vi "control loop bookkeeping.vi"(6 "worker pool reference":T2, 8 "engine error in":errorcluster, 9 "status reporting in":T18={"late? index (bool)"=-1, "late count index (U32)"=-1, "dt (ns) index (U64)"=-1}, 10 "time data in":T1, 11 "control loop data in":T5 {"module information"."GUID"."Lo" format="%.0x"; "module information"."GUID"."Hi" format="%.0x"}) -> (0 "engine error out":errorcluster, 1 "safe state?":bool, 2 "time data out":T1, 3 "control loop data out":T5 {"module information"."GUID"."Lo" format="%.0x"; "module information"."GUID"."Hi" format="%.0x"})   [LabVIEW 2013, in "main engine.lvlib"]
doc: "This VI writes to any of the timing or error tags that have been configured based on the results of this iteration of the loop."
uses:
  main engine.lvlib
  status reporting data.ctl
  control loop data.ctl
  <vilib>/NI/Tag Bus/table/data table.ctl
  engine run schedule.ctl
  engine decimation schedule.ctl
  full module data.ctl
  <vilib>/NI/Tag Bus Module Framework/runtime/TBM module execution interface.lvclass
  module run state.ctl
  async executor/asynchronous executor reference.ctl
  async executor/message to executor.ctl
  Runtime/async command notification.ctl
  Runtime/async error info.ctl
  <vilib>/NI/Tag Bus Module Framework/runtime/error classification.ctl
  <vilib>/NI/Tag Bus Module Framework/module configuration/TBM module configuration.lvclass
  <vilib>/NI/Configuration Framework/serializable configuration/Numeric GUID.ctl
  module method data.ctl
  <vilib>/NI/Tag Bus/table/transfer specification.ctl
  <vilib>/NI/Tag Bus/tag/Data Type.ctl
  fault handling spec.ctl
  Configuration/Error Actions.ctl
  worker library/worker comms.ctl
  worker library/worker commands.ctl
  worker library/request fifos.ctl
  worker library/recovery request.ctl
  worker library/rt fault.ctl
  worker library/response fifos.ctl
  worker library/recovery response.ctl
  <vilib>/NI/Module Execution Interface/Engine Runtime/Fault.ctl
  time information.ctl
  <vilib>/NI/Tag Bus/table/write data element.vi
  <vilib>/NI/Tag Bus/table/data polymorphs/write one/write I32.vi
  perform asynchronous fault handling.vi
  perform fault handling.vi
  <vilib>/NI/Tag Bus/table/data polymorphs/write one/write Boolean.vi
  <vilib>/NI/Tag Bus/table/data polymorphs/write one/write U32.vi
  <vilib>/NI/Tag Bus/table/data polymorphs/write one/write U64.vi
  worker library/request recovery.vi
  worker library/request fault.vi
  rt swap object in dvr.vi
  <vilib>/NI/Tag Bus/table/data table.lvlib
  <vilib>/NI/Tag Bus/tag/tag descriptor.lvclass
  Configuration/Standard Engine Configuration.lvclass
  async executor/async executor.lvlib
  <vilib>/NI/Configuration Framework/serializable configuration/NISE_CEF_serializable configuration.lvclass
  worker library/worker pool.lvlib
  <vilib>/NI/Module Execution Interface/Engine Runtime/Engine Runtime Interface.lvclass
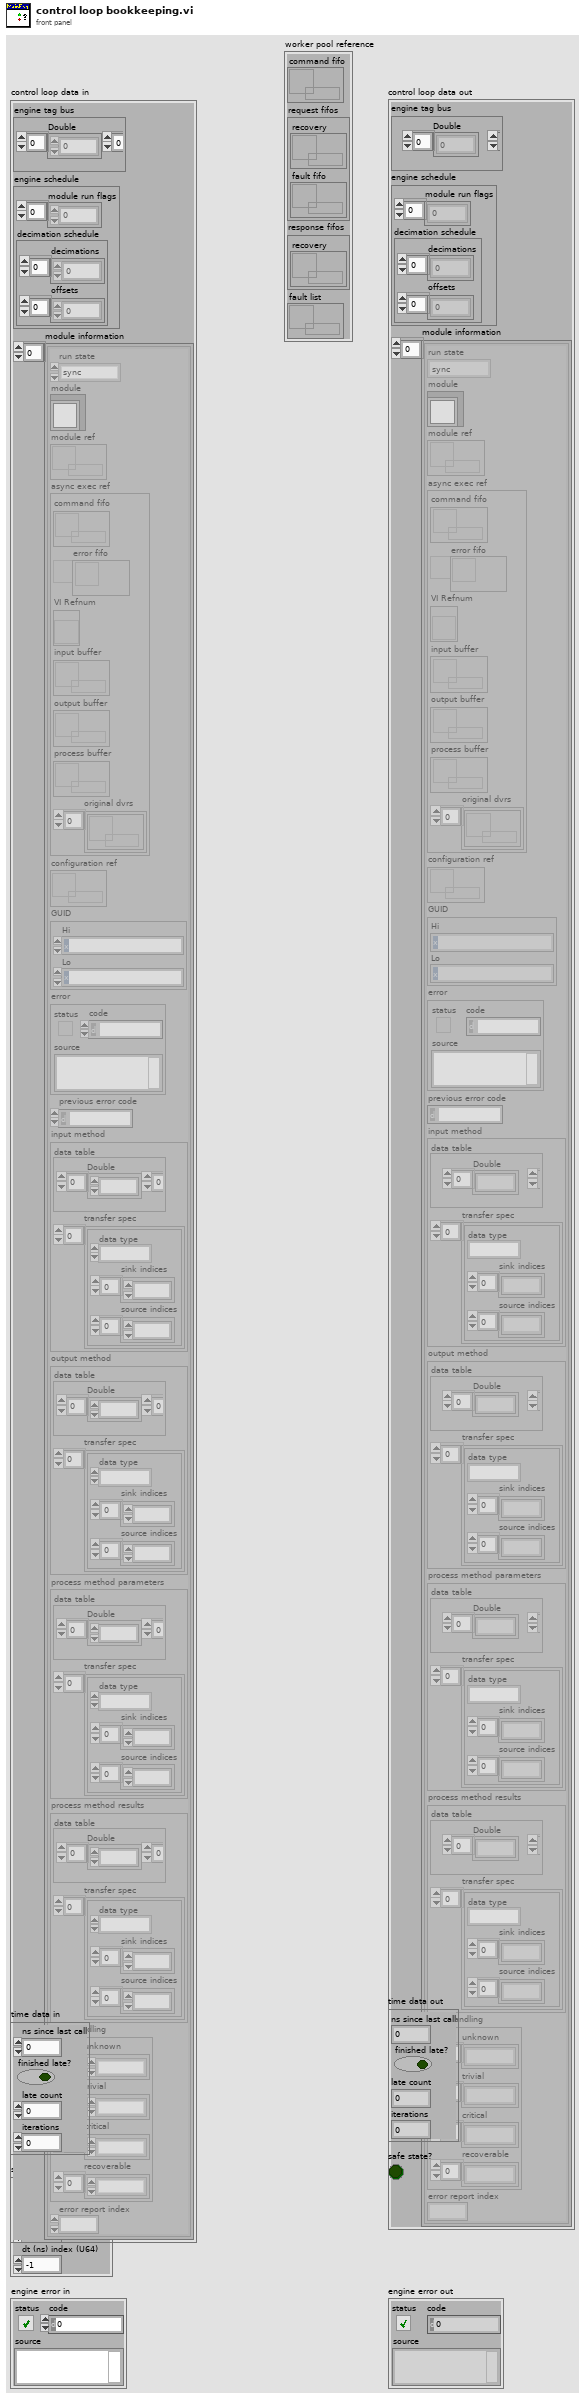
[diagram p1: front panel]
types:
  T1 = typedef "main engine.lvlib/time information.ctl" = cluster{"ns since last call":u64, "finished late?":bool, "late count":u32, "iterations":u64}
  T2 = typedef "worker pool.lvlib/worker comms.ctl" = cluster{"command fifo":refnum<k33>, "request fifos":T3, "response fifos":T4, "fault list":refnum<data-value>}
  T3 = typedef "worker pool.lvlib/request fifos.ctl" = cluster{"recovery":refnum<k33>, "fault fifo":refnum<k33>}
  T4 = typedef "worker pool.lvlib/response fifos.ctl" = cluster{"recovery":refnum<k33>}
  T5 = typedef "main engine.lvlib/control loop data.ctl" = cluster{"engine tag bus":T6, "engine schedule":T7, "module information":T9[]}
  T6 = typedef "tag bus.lvlib/data table.lvlib/data table.ctl" = cluster{"Double":dbl[], "Single":sgl[], "I64":i64[], "I32":i32[], "I16":i16[], "I8":i8[], "U64":u64[], "U32":u32[], "U16":u16[], "U8":u8[], "Boolean":bool[], "String":string[], "Array of Double":cluster{"DBL Array":dbl[]}[], "Array of Single":cluster{"SGL Array":sgl[]}[], "Array of I64":cluster{"I64 Array":i64[]}[], "Array of I32":cluster{"I32 Array":i32[]}[], "Array of I16":cluster{"I16 Array":i16[]}[], "Array of I8":cluster{"I8 Array":i8[]}[], "Array of U64":cluster{"U64 Array":u64[]}[], "Array of U32":cluster{"U32 Array":u32[]}[], "Array of U16":cluster{"U16 Array":u16[]}[], "Array of U8":cluster{"U8 Array":u8[]}[], "Array of Boolean":cluster{"Boolean Array":bool[]}[], "Array of String":cluster{"String Array":string[]}[]}
  T7 = typedef "main engine.lvlib/engine run schedule.ctl" = cluster{"module run flags":u8[], "decimation schedule":T8}
  T8 = typedef "main engine.lvlib/engine decimation schedule.ctl" = cluster{"decimations":u16[], "offsets":u16[]}
  T9 = typedef "main engine.lvlib/full module data.ctl" = cluster{"run state":T10, "module":refnum<class "TBM module execution interface.lvclass">, "module ref":refnum<data-value>, "async exec ref":T11, "configuration ref":refnum<data-value>, "GUID":T12, "error":errorcluster, "previous error code":i32, "input method":T13, "output method":T13, "process method parameters":T13, "process method results":T13, "fault handling":T16, "error report index ":i32}
  T10 = typedef "main engine.lvlib/module run state.ctl" = enum16{"sync", "async"}
  T11 = typedef "async executor.lvlib/asynchronous executor reference.ctl" = cluster{"command fifo":refnum<k33>, "error fifo":refnum<k33>, "VI Refnum":refnum<vi>, "input buffer":refnum<k33>, "output buffer":refnum<k33>, "process buffer":refnum<k33>, "original dvrs":refnum<data-value>[]}
  T12 = typedef "NISE_CEF_serializable configuration.lvclass/Numeric GUID.ctl" = cluster{"Hi":u64, "Lo":u64}
  T13 = typedef "main engine.lvlib/module method data.ctl" = cluster{"data table":T6, "transfer spec":T14[]}
  T14 = typedef "tag bus.lvlib/data table.lvlib/transfer specification.ctl" = cluster{"data type":T15, "sink indices":i32[], "source indices":i32[]}
  T15 = typedef "tag bus.lvlib/tag descriptor.lvclass/Data Type.ctl" = enum16{"Double", "Single", "I64", "I32", "I16", "I8", "U64", "U32", "U16", "U8", "Boolean", "String", "Array of Double", "Array of Single", "Array of I64", "Array of I32", "Array of I16", "Array of I8", "Array of U64", "Array of U32", "Array of U16", "Array of U8", "Array of Boolean", "Array of String"}
  T16 = typedef "main engine.lvlib/fault handling spec.ctl" = cluster{"unknown":T17[], "trivial":T17[], "critical":T17[], "recoverable":T17[]}
  T17 = typedef "Standard Engine Configuration.lvclass/Error Actions.ctl" = enum16{"Clear", "Notify", "Stop Component", "Stop Engine", "Safe State", "Attempt Recovery"}
  T18 = typedef "main engine.lvlib/status reporting data.ctl" = cluster{"late? index (bool)":i32, "late count index (U32)":i32, "dt (ns) index (U64)":i32}
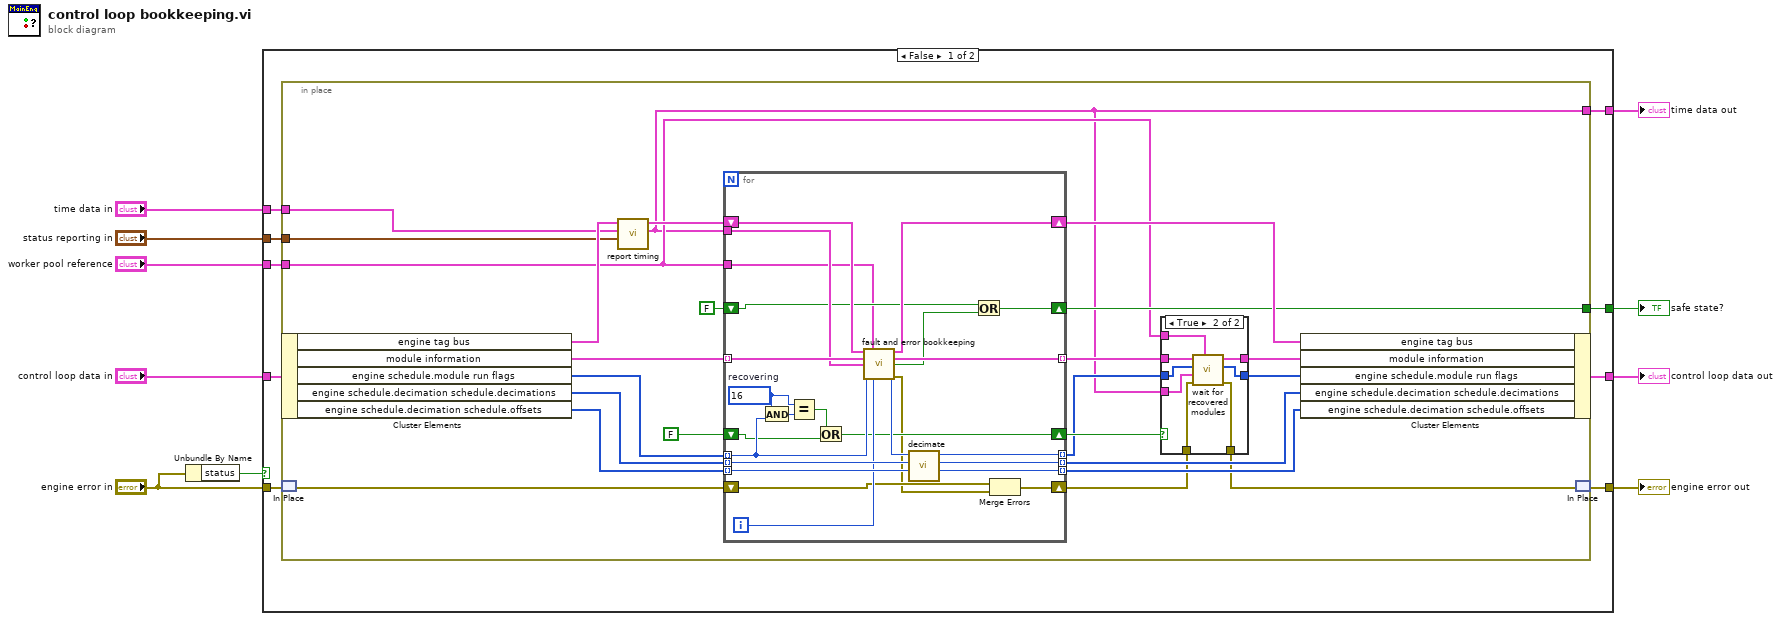
[diagram p0: block diagram]
diagram:
  n1 = Unbundle By Name("engine error in") -> ("status"=w1:bool)
  n2 = case shown="False" w1 {
    tunnel: "control loop data in" -> [w19 w80]
    tunnel: [w18 w80] -> w9
    tunnel: "engine error in" -> [w17 w81]
    tunnel: [w16 w81] -> w8
    tunnel: "status reporting in" -> [w15 _]
    tunnel: "worker pool reference" -> [w14 _]
    tunnel: [w13 _] -> w5
    tunnel: [w12 w82] -> w4
    tunnel: "time data in" -> [w11 w82]
    frame False {
      n3 = in-place {
        in-place-border: [w21] -> w12
        in-place-border: w11 -> [w35]
        in-place-border: w15 -> [w31]
        in-place-border: w14 -> [w24]
        in-place-border: [w32] -> w13
        n4 = in-place-cluster #1(w19) -> ("engine tag bus"=w36:T6, "module information"=w42:T9[], "engine schedule.module run flags"=w41:u8[], "engine schedule.decimation schedule.decimations"=w39:u16[], "engine schedule.decimation schedule.offsets"=w34:u16[])
        n5 = in-place-match #2(w17) -> (w38:errorcluster)
        n6 = call "report timing.vi"("status reporting tags"=w31, "time data in"=w35, "engine tag bus"=w36) -> ("time data out"=w21:T1, "engine data out"=w37:T6)  [unwired: 7 in]
        n7 = for {
          shift-right: [w72] -> w43
          shift-left: w37 -> [w73]
          tunnel: w42 -> [w70] mode=indexing
          tunnel: w41 -> [w64] mode=indexing
          tunnel: [w79] -> w26 mode=indexing
          tunnel: [w78] -> w40 mode=indexing
          tunnel: [w77] -> w33 mode=indexing
          tunnel: w39 -> [w75] mode=indexing
          tunnel: w34 -> [w74] mode=indexing
          shift-right: [w56] -> w23
          shift-left: w38 -> [w58]
          tunnel: w24 -> [w55]
          tunnel: [w71] -> w28 mode=indexing
          tunnel: w21 -> [w68]
          shift-right: [w62] -> w29
          shift-left: FALSE -> [w61]
          shift-right: [w60] -> w32
          shift-left: FALSE ("safe state?") -> [w59]
          i -> [w67]
          w66 = u8 16  # recovering
          n8 = And(x=w66, y=w64) -> (x .and. y?=w65:u8)
          n9 = Equal?(x=w66, y=w65) -> (x = y?=w63:bool)
          n10 = Or(x=w63, y=w61) -> (x .or. y?=w62:bool)
          n11 = call "fault and error bookkeeping.vi"("data table in"=w73, "worker pool reference"=w55, "module data"=w70, "time data in"=w68, "run flags in"=w64, "module index"=w67) -> ("data table out"=w72:T6, "module data out"=w71:T9, "safe state?"=w69:bool, "run flags out"=w76:u8, "engine error out"=w57:errorcluster)  [unwired: 5 in]
          n12 = call "decimate.vi"("offset"=w74, "decimation"=w75, "run flags"=w76) -> ("new offset"=w77:u16, "decimation out"=w78:u16, "run flags out"=w79:u8)  [unwired: 6 in]
          n13 = Or(x=w59, y=w69) -> (x .or. y?=w60:bool)
          n14 = Merge Errors(w58, w57) -> (w56:errorcluster)
        }
        n15 = case shown="True" w29 {
          tunnel: w28 -> [w46 w53]
          tunnel: [w46 w54] -> w27
          tunnel: w26 -> [w45 w52]
          tunnel: [w45 w51] -> w25
          tunnel: w24 -> [_ w47]
          tunnel: w23 -> [w44 w50]
          tunnel: [w44 w49] -> w22
          tunnel: w21 -> [_ w48]
          frame False {
          }
          frame True {
            n16 = call "wait for recovered modules.vi"("worker pool reference"=w47, "error in"=w50, "time data in"=w48, "run flags in"=w52, "modules in"=w53) -> ("error out"=w49:errorcluster, "run flags out"=w51:u8[], "modules out"=w54:T9[])  [unwired: 4 in]
          }
        }
        n17 = in-place-cluster #1("engine tag bus"=w43, "module information"=w27, "engine schedule.module run flags"=w25, "engine schedule.decimation schedule.decimations"=w40, "engine schedule.decimation schedule.offsets"=w33) -> (w18:T5)
        n18 = in-place-match #2(w22) -> (w16:errorcluster)
      }
    }
    frame True {
    }
  }
  "control loop data out" <- w9
  "engine error out" <- w8
  "safe state?" <- w5
  "time data out" <- w4
